vi "sym matrix to compact form.vi"(10 "Preallocated Compact Form":dbl[](array[numeric]), 11 "Symmetric Matrix":T1) -> (0 "error":i32, 2 "Compact Form":dbl[](array[numeric]))   [LabVIEW 2017, in "NI_AALPro.lvlib"]
uses:
  NI_AALPro.lvlib
  RealMatrix.ctl
  lvanlys.dll
  NI_Matrix.lvlib
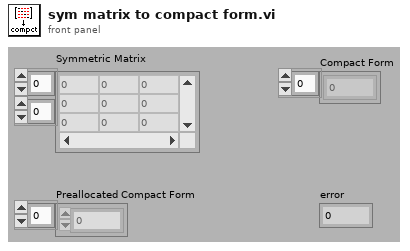
[diagram p1: front panel]
types:
  T1 = typedef "NI_Matrix.lvlib/RealMatrix.ctl" = dbl[][]
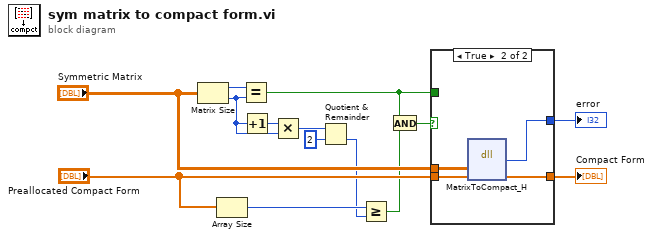
[diagram p0: block diagram]
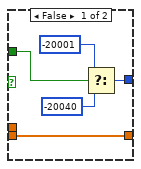
[diagram p2: hidden frame]
diagram:
  n1 = Matrix Size(0:"Symmetric Matrix") -> (1:w12:i32, 2:w1:i32)
  n2 = Array Size(array="Preallocated Compact Form") -> (size(s)=w7:i32)
  n3 = Equal?(x=w12, y=w1) -> (x = y?=w2:bool)
  n4 = Increment(x=w1) -> (x+1=w11:i32)
  n5 = Multiply(x=w11, y=w1) -> (x*y=w10:i32)
  n6 = Quotient & Remainder(x=w10, y=2) -> (floor(x/y)=w6:i32)  [unwired: 1 out]
  n7 = Greater Or Equal?(x=w7, y=w6) -> (x >= y?=w5:bool)
  n8 = And(x=w2, y=w5) -> (x .and. y?=w4:bool)
  n9 = case shown="True" w4 {
    tunnel: "Preallocated Compact Form" -> [w19 w23]
    tunnel: [w19 w22] -> w14
    tunnel: "Symmetric Matrix" -> [_ w21]
    tunnel: [w17 w20] -> w3
    tunnel: w2 -> [w18 _]
    frame False {
      n10 = Select(t=-20001 ("error"), s=w18, f=-20040 ("error")) -> (s? t:f=w17:i32)
    }
    frame True {
      n11 = dll-call lib="C:/Program Files/National Instruments/LabVIEW 2017/resource/lvanlys.*" fn="MatrixToCompact_H"("matrixH"=w21, "aH"=w23) -> ("return type"=w20:i32, "aH"=w22:dbl[])  [unwired: 4 in, 2 out]
    }
  }
  "Compact Form" <- w14
  "error" <- w3
